vi "Synchronised one pulse signal generation and acquisition.vi"() -> ()   [LabVIEW 2010]
doc: "This example shows how to acquire 16k samples of signal on fast analog inputs. Signal will be acquired simultaneously with generated signal. Time length of the acquired signal depends on the time scale of a buffer that can be set with a decimation factor. Decimations and time scales of a buffer are given in the table below. Voltage range of fast analog inputs on the Red Pitaya depends on gain setting that can be set by jumpers. HV setting is for input range to ±20V, while LV sets input range to ±1V."
uses:
  RedPitaya.lvlib
panel:
  in  "Trigger Level (0 mV)":i32=50
  in  "Delay (# Samples)":i32
  in  "Averaging":enum16{"None", "AVG ON", "AVG OFF"}(ring)
  in  "Decimation":u32(ring)=1 items=["65536"=65536, "8192"=8192, "1024"=1024, "64"=64, "8"=8, "1"=1]
  in  "Total Time of One Burst":i32=-1
  in  "Number of repeated Bursts":string
  in  "Number of generated Signals / Burst":string="1"
  in  "Duty Cycle":i32=-1 min=-1 max=100
  in  "Phase":i32=361
  in  "DC Offset":dbl=2.0
  in  "Frequency (1000 Hz)":i32=50000
  in  "Amplitude":dbl=1.0
  in  "Waveform Function":u16(ring)=1 items=["", "Sine", "Square", "Triangle", "Sawtooth UP", "Sawtooth Down", "PWM"]
  in  "Channel (1|2)":u16(ring)=1 items=["Channel 1"=1, "Channel 2"=2]
  in  "IP address":string="192.168.1.100"
  out "Waveform Graph":dbl[](graph)
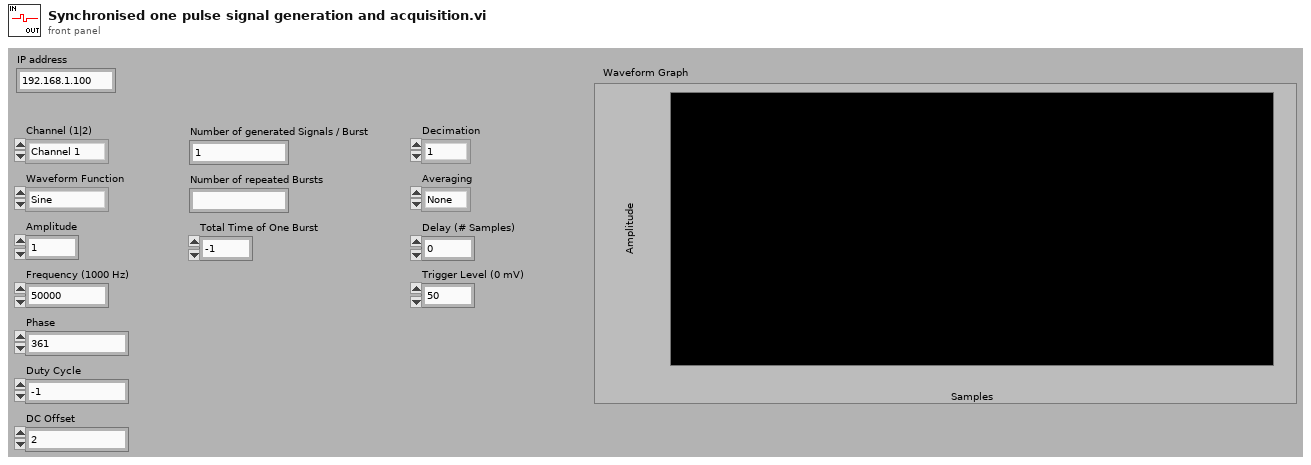
[diagram p1: front panel]
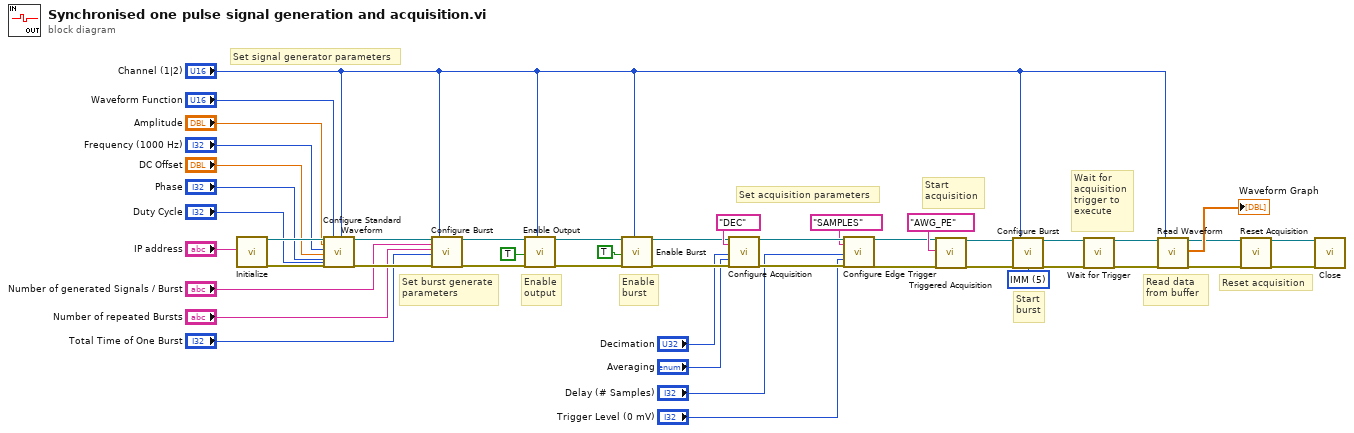
[diagram p0: block diagram]
diagram:
  w19 = u16 5 items=["", "EXT_PE", "EXT_NE", "INT", "GATED", "IMM"] ("Trigger Source")
  # "Reset acquisition"
  # "Read data\nfrom buffer"
  # "Wait for\nacquisition\ntrigger to \nexecute"
  # "Start\nburst"
  # "Start\nacquisition"
  # "Set acquisition parameters"
  # "Enable\nburst"
  # "Enable\noutput"
  # "Set burst generate\nparameters"
  # "Set signal generator parameters"
  n1 = call "Initialize.vi"("IP address"="IP address") -> ("RedPitaya TCP Connection"=w41:refnum<k5>, "error out"=w40:errorcluster)  [unwired: 17 in]
  n2 = call "Configure Standard Waveform.vi"("RedPitaya connection in"=w41, "Amplitude"="Amplitude", "Frequency"="Frequency (1000 Hz)", "DC Offset"="DC Offset", "Phase"="Phase", "error in"=w40, "Channel #"="Channel (1|2)", "Duty Cycle"="Duty Cycle", "Waveform Function"="Waveform Function") -> ("RedPitaya connection out"=w35:refnum<k5>, "error out"=w34:errorcluster)  [unwired: 9 in]
  n3 = call "Configure Burst.vi"("RedPitaya connection in"=w35, "Number of generated Signals / Burst"="Number of generated Signals / Burst", "Number of repeated Bursts"="Number of repeated Bursts", "Total time of One Burst"="Total Time of One Burst", "error in"=w34, "Channel #"="Channel (1|2)") -> ("RedPitaya connection out"=w33:refnum<k5>, "error out"=w32:errorcluster)  [unwired: 12 in]
  n4 = call "Enable Output.vi"("RedPitaya connection in"=w33, "Generation (T: Enable)"=TRUE, "error in"=w32, "Channel #"="Channel (1|2)") -> ("RedPitaya connection out"=w25:refnum<k5>, "error out"=w24:errorcluster)  [unwired: 14 in]
  n5 = call "Enable Burst.vi"("RedPitaya connection in"=w25, "Generation (T: Enable)"=TRUE, "error in"=w24, "Channel #"="Channel (1|2)") -> ("RedPitaya connection out"=w27:refnum<k5>, "error out"=w26:errorcluster)  [unwired: 14 in]
  n6 = call "Configure Acquisition.vi"("RedPitaya connection in"=w27, "Decimation/Sampling Rate"="DEC", "Decimation"="Decimation", "Averaging"="Averaging", "error in"=w26) -> ("RedPitaya connection out"=w38:refnum<k5>, "error out"=w37:errorcluster)  [unwired: 13 in]
  n7 = call "Configure Edge Trigger.vi"("RedPitaya connection in"=w38, "Trigger Delay mode"="SAMPLES", "Delay (# Samples)"="Delay (# Samples)", "Trigger Level (0 mV)"="Trigger Level (0 mV)", "error in"=w37) -> ("RedPitaya connection out"=w44:refnum<k5>, "error out"=w43:errorcluster)  [unwired: 13 in]
  n8 = call "Triggered Acquisition.vi"("RedPitaya TCP connection in"=w44, "Trigger Mode"="AWG_PE", "error in"=w43) -> ("RedPitaya TCP connection out"=w23:refnum<k5>, "error out"=w22:errorcluster)  [unwired: 15 in]
  n9 = call "Configure Burst.vi"("RedPitaya connection in"=w23, "Trigger Source"=w19, "error in"=w22, "Channel #"="Channel (1|2)") -> ("RedPitaya connection out"=w21:refnum<k5>, "error out"=w20:errorcluster)  [unwired: 14 in]
  n10 = call "Wait for Trigger.vi"("RedPitaya TCP connection in"=w21, "error in"=w20) -> ("RedPitaya TCP connection out"=w30:refnum<k5>, "error out"=w29:errorcluster)  [unwired: 16 in]
  n11 = call "Read Waveform.vi"("RedPitaya TCP Connection in"=w30, "error in"=w29, "Channel #"="Channel (1|2)") -> ("RedPitaya TCP Connection out"=w18:refnum<k5>, "Measurement Array"=→"Waveform Graph":dbl[], "error out"=w15:errorcluster)  [unwired: 14 in]
  n12 = call "Reset Acquisition.vi"("RedPitaya connection in"=w18, "error in"=w15) -> ("RedPitaya connection out"=w17:refnum<k5>, "error out"=w16:errorcluster)  [unwired: 16 in]
  n13 = call "Close.vi"("connection ID"=w17, "error in"=w16) -> ()  [unwired: 17 in, 1 out]
